vi "Initialize.vi"(8 "error in (no error)":errorcluster, 9 "Reset Device (T:Reset Device)":bool=TRUE, 10 "ID Query (F:Skip Query)":bool, 11 "VISA resource name":refnum<visa-resource-name>) -> (0 "error out":errorcluster, 3 "VISA resource name out":refnum<visa-resource-name>)   [LabVIEW 2011, in "Agilent 4194.lvlib"]
doc: "This function performs the following initialization actions:\n\n- Opens a session to the Default Resource Manager resource and a session to the specified device using the interface and address specified in the Resource_Name control.\n\n- Performs an identification query on the Instrument.\n\n- Resets the instrument to a known state.\n\n- Sends initialization commands to the instrument that set any necessary programmatic variables such as Headers Off, Short Command form, and Data Transfer Binary to the state necessary for the operation of the instrument driver.\n\n- Returns an Instrument Handle which is used to differentiate between different sessions of this instrument driver.\n\n- Each time this function is invoked a Unique Session is opened. It is possible to have more than one session open for the same resource.\n\nNotes:\n\n(1) This instrument does not support an ID Query and this VI will return an warning if the 'ID Query' control is set to \"T\"-Do Query."
uses:
  <instrlib>/Agilent 4194/Agilent 4194.lvlib
panel:
  # "© 2005 National Instruments.  ALL RIGHTS RESERVED."
  # "Do Query\nSkip Query"
  # "Reset Device\nDon't Reset"
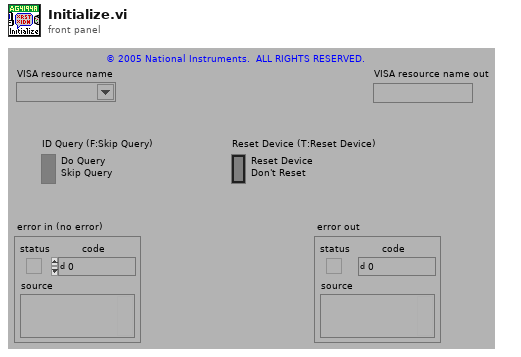
[diagram p1: front panel]
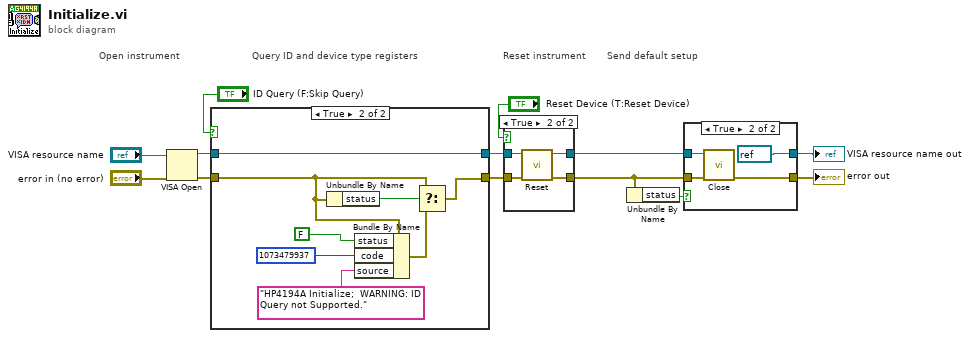
[diagram p0: block diagram]
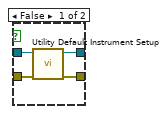
[diagram p3: hidden frame]
diagram:
  # "Send default setup"
  # "Query ID and device type registers"
  # "Reset instrument"
  # "Open instrument"
  n1 = VISA Open(error in (no error)="error in (no error)", VISA resource name="VISA resource name") -> (VISA resource name=w11:refnum<visa-resource-name>, error out=w10:errorcluster)  [unwired: 3 in]
  n2 = case shown="True" "ID Query (F:Skip Query)" {
    tunnel: [w14 w17] -> w12
    tunnel: [w15 w16] -> w13
    tunnel: w11 -> [w15 w16]
    tunnel: w10 -> [w14 w18]
    frame False {
    }
    frame True {
      n3 = Unbundle By Name(w18) -> ("status"=w22:bool)
      n4 = Bundle By Name(cluster=w18, "status"=FALSE, "code"=1073479937, "source"="HP4194A Initialize;  WARNING: ID Query not Supported.") -> (w23:errorcluster)
      n5 = Select(t=w18, s=w22, f=w23) -> (s? t:f=w17:errorcluster)
    }
  }
  n6 = case shown="True" "Reset Device (T:Reset Device)" {
    tunnel: w12 -> [w26 w29]
    tunnel: [w25 w28] -> w1
    tunnel: w13 -> [w27 w31]
    tunnel: [w24 w30] -> w2
    frame False {
      n7 = call <instrlib>:"Utility Default Instrument Setup.vi"("error in (no error)"=w26, "VISA resource name"=w27) -> ("error out"=w25:errorcluster, "VISA resource name out"=w24:refnum<visa-resource-name>)  [unwired: 8 in]
    }
    frame True {
      n8 = call <instrlib>:"Reset.vi"("error in (no error)"=w29, "VISA resource name"=w31) -> ("error out"=w28:errorcluster, "VISA resource name out"=w30:refnum<visa-resource-name>)  [unwired: 8 in]
    }
  }
  n9 = Unbundle By Name(w1) -> ("status"=w9:bool)
  n10 = case shown="True" w9 {
    tunnel: [w32 w35] -> w3
    tunnel: [w33 refnum<visa-resource-name> refnum ("VISA resource name out")] -> w4
    tunnel: w2 -> [w33 w36]
    tunnel: w1 -> [w32 w37]
    frame False {
    }
    frame True {
      n11 = call <instrlib>:"Close.vi"("error in (no error)"=w37, "VISA resource name"=w36) -> ("error out"=w35:errorcluster)  [unwired: 9 in]
    }
  }
  "error out" <- w3
  "VISA resource name out" <- w4
